vi "PDF Protokoll EPA1065_305 ARN.vi"(8 "error in (no error)":errorcluster caption="Fehler (Eingang, kein Fehler)", 11 "Tabelle":string[][](table)) -> (0 "error out":errorcluster caption="Fehler (Ausgang)")   [LabVIEW 2020, in "EPA 1065.lvlib" / "ARN Test 1065-305.lvlib"]
uses:
  ARN Test 1065-305.lvlib
  T90 1065-308/Ergebnis.ctl
  Seiten/FT-IR/FGV FT-IR Gasliste Aktionen.ctl
  Seiten/FT-IR/FGV FT-IR Aktionen.ctl
  Aktion FGV ARN Daten.ctl
  Aktion FGV Protokoll.ctl
  Seiten/System Einstellungen V2/Aktioen FGV System Konstanten.ctl
  <vilib>/Utility/miscctls.llb/LVPrintingMarginsTypeDef.ctl
  Allgemein/allgemeine Sub-VIs.lvlib
  Seiten/FT-IR/FT-IR.lvlib
  Seiten/System Einstellungen V2/System Einstellungen V2.lvlib
  T90 1065-308/T90 Test 1065-308.lvlib
panel:
  out "Versa Serial number:":string caption="Seriennummer:"
  out "Anlage:":string
  out "Einheit Noise 2":string
  out "Einheit Wiederh. 2":string
  out "Einheit Genauigkeit 2":string
  out "Einheit Noise":string
  out "Einheit Wiederh.":string
  out "Ergebnis 3":T1
  out "Ergebnis 2":T1
  out "Ergebnis 1":T1
  out "Rauschen":string
  out "Rauschen Grenze":string caption="Rauschen:"
  out "Wiederholgenauigkeit":string
  out "Genauigkeit":string
  out "Wiederholgenauigkeit Grenze":string caption="Wiederholgenauigkeit:"
  out "Genauigkeit Grenze":string caption="Genauigkeit:"
  out "Einheit Genauigkeit":string
  out "Tabelle":string[][](table)
  out "Methode (Recipe):":string caption="Methode (Rezept):"
  out "Date & Time:":string caption="Datum & Zeit:"
  out "Accuracy:":string caption="Genauigkeit:"
  out "Gas Bottle Nr.:":string caption="Gasflaschen Nr.:"
  out "T90 Result":waveform(dbl)(graph) caption="T90"
  out "Ergebnis:":string
  out "Konzentration:":string caption="Sollwert:"
  out "Komponente:":string
  out "Bearbeiter:":string
  out "Serial number:":string caption="Seriennummer:"
  out "Messgerät:":string
  # "ANR EPA § 1065.305"
  # "Grenzen"
  # "Ergebnis"
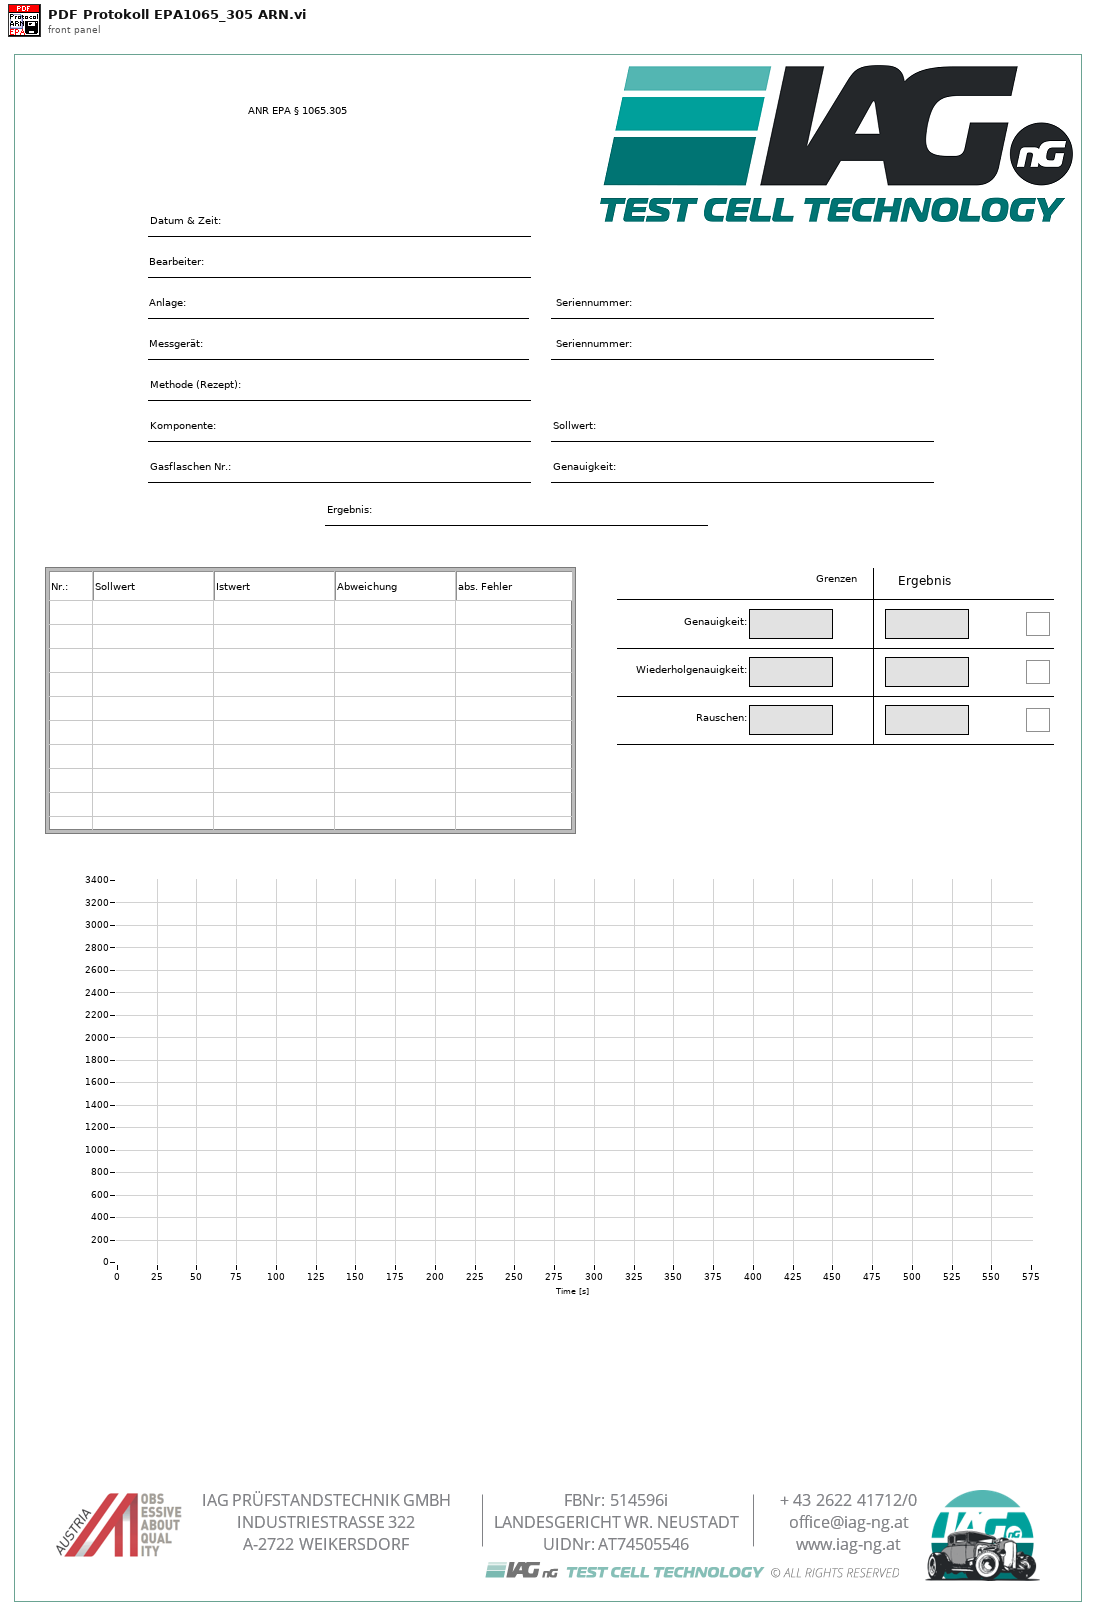
[diagram p1: front panel]
types:
  T1 = typedef "EPA 1065.lvlib/T90 Test 1065-308.lvlib/Ergebnis.ctl" = bool
  T2 = typedef "EPA 1065.lvlib/ARN Test 1065-305.lvlib/Aktion FGV ARN Daten.ctl" = enum16{"Lesen", "laden", "speichern", "ARN Daten", "Rohdaten", "Rohdaten löschen", "Zeitstempel", "SNR Ergebnis"}
  T3 = typedef "FT-IR.lvlib/FGV FT-IR Aktionen.ctl" = enum16{"lesen", "NOG setzen", "NOS setzen", "Initialisieren", "speichern", "ALLES setzen", "FT-IR Spektrum loggen", "Komm Stoppen", "Spektrum LogKonfig"}
  T4 = typedef "FT-IR.lvlib/FGV FT-IR Gasliste Aktionen.ctl" = enum16{"lesen", "Gasliste FT-IR", "Gasliste ausgelesen", "laden", "speichern", "löschen"}
  T5 = typedef "System Einstellungen V2.lvlib/Aktioen FGV System Konstanten.ctl" = enum16{"lesen", "laden", "speichern", "Sprache"}
  T6 = typedef "EPA 1065.lvlib/ARN Test 1065-305.lvlib/Aktion FGV Protokoll.ctl" = enum16{"lesen", "schreiben", "Graph"}
  T7 = enum32{"Portrait", "Landscape", "Rotated Portrait", "Rotated Landscape"}
  T8 = typedef "LVPrintingMarginsTypeDef.ctl" = cluster{"Top":sgl, "Left":sgl, "Bottom":sgl, "Right":sgl, "Measurement System":enum8{"Inches", "cm"}}
  T9 = typedef "EPA 1065.lvlib/ARN Test 1065-305.lvlib/Allgemeine Einstellungen.ctl" = cluster{"Bearbeiter:":string, "Analysator":T10, "Komponente:":u16, "Gasflaschen Nr.:":string, "Accuracy":dbl, "Sollwert":dbl, "Modus":T11, "Pfad:":path, "Textname:":string, "CG Aufschaltzeit:":dbl, "Einheit":string, "N2 Aufschaltzeit:":dbl, "Gasflasche":T12, "Konfig Gasflasche":T13}
  T10 = typedef "System Einstellungen V2.lvlib/Analysatoren.ctl" = string
  T11 = typedef "EPA 1065.lvlib/T90 Test 1065-308.lvlib/Modus.ctl" = u16
  T12 = typedef "System Einstellungen V2.lvlib/Gasflasche Auswahl.ctl" = u16
  T13 = typedef "System Einstellungen V2.lvlib/Konfig Gasflasche.ctl" = bool
  T14 = typedef "String - Ausgabefeld.ctl" = string
  T15 = cluster{"Modell":string, "ProjektNummer":string, "Software Version":string, "Seriennummer":string}
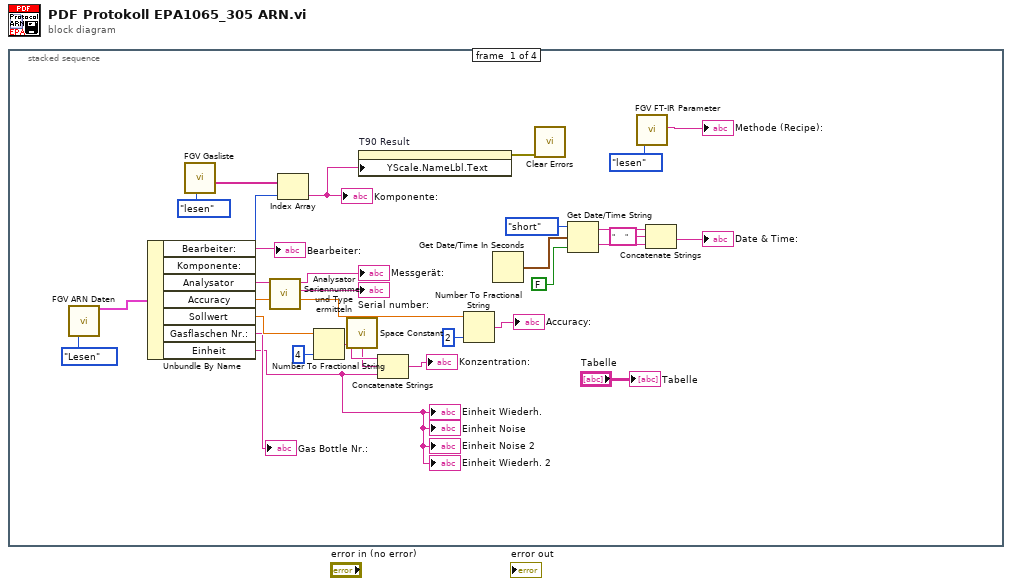
[diagram p0: block diagram]
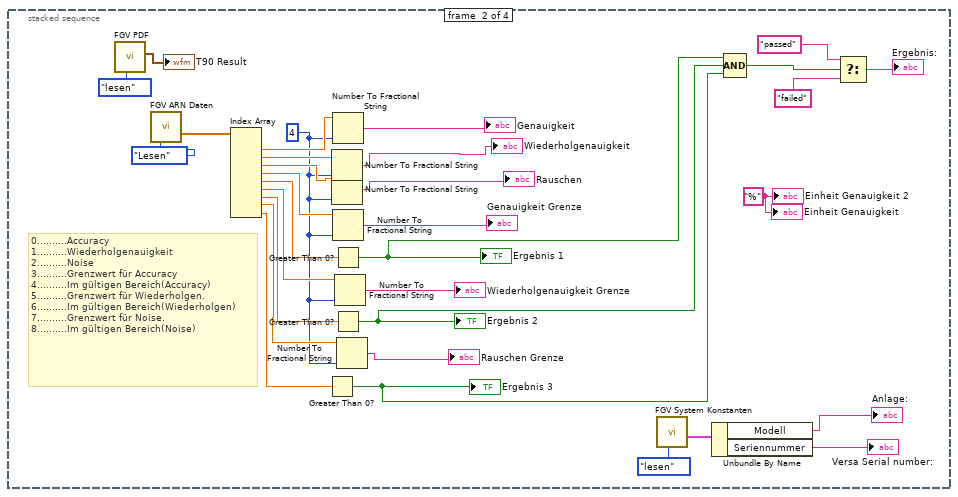
[diagram p2: hidden frame]
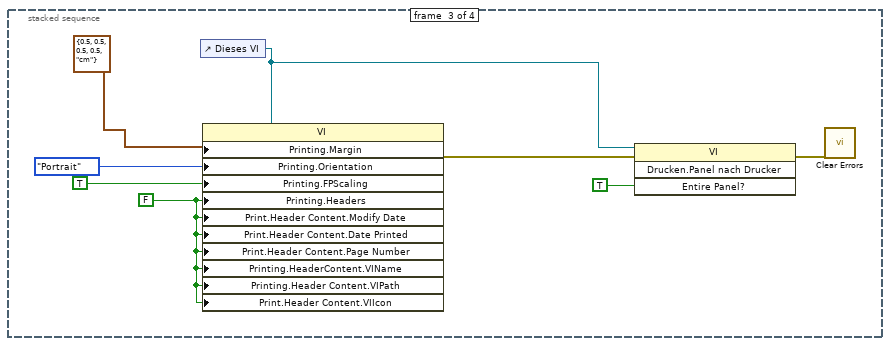
[diagram p3: hidden frame]
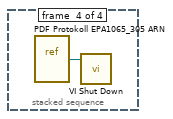
[diagram p4: hidden frame]
diagram:
  n1 = stacked-sequence {
    frame #0 {
      n2 = call "FGV ARN Daten.vi"("Aktion"=Aktion_FGV_ARN_Daten."Lesen") -> ("ARN Konfig Daten"=w6:T9)  [unwired: 9 in, 5 out]
      n3 = Unbundle By Name(w6) -> ("Bearbeiter:"=→"Bearbeiter:":string, "Komponente:"=w21:u16, "Analysator"=w3:T10, "Accuracy"=w18:dbl, "Sollwert"=w14:dbl, "Gasflaschen Nr.:"=→"Gas Bottle Nr.:":string, "Einheit"=w4:string)
      "Einheit Wiederh. 2" <- w4
      "Einheit Noise 2" <- w4
      "Einheit Noise" <- w4
      "Einheit Wiederh." <- w4
      n4 = call "FGV Gasliste.vi"("Aktionen"=FGV_FT-IR_Gasliste_Aktionen."lesen") -> ("Aktuelle Gasliste gesamt"=w22:T14[])  [unwired: 8 in, 2 out]
      n5 = call "Analysator Seriennummer und Type ermitteln.vi"("Analysator"=w3) -> ("Type"=→"Serial number:":string, "Name für Protokoll"=→"Messgerät:":string)  [unwired: 8 in, 1 out]
      n6 = Index Array(array=w22, index=w21) -> (element=w11:T14)
      "Komponente:" <- w11
      n7 = Number To Fractional String(number=w14, precision (6)=i16 4 ("Genauigkeit (6)")) -> (F-format string=w10:string)  [unwired: 2 in]
      n8 = call <vilib>:"Space Constant.vi"() -> ("String"=w8:string)
      n9 = property on="T90 Result" class="SVGraph (strikt)"("YScale.NameLbl.Text"=w11) -> (error out=w12:errorcluster)  [unwired: 2 in, 1 out]
      n10 = Concatenate Strings(w10, w8, w4) -> (→"Konzentration:":string)
      n11 = Number To Fractional String(number=w18, precision (6)=i16 2 ("Genauigkeit (6)")) -> (F-format string=→"Accuracy:":string)  [unwired: 2 in]
      n12 = Get Date/Time In Seconds() -> (seconds since 1Jan1904=w31:timestamp)
      n13 = call <vilib>:"Clear Errors.vi"("error in (no error)"=w12) -> ()  [unwired: 5 in, 2 out]
      n14 = Get Date/Time String(date format (0)=enum16{"short", "long", "abbreviated"}."short" ("Datumsformat (0)"), seconds (now)=w31, want seconds? (F)=FALSE ("Angabe von Sekunden? (F)")) -> (date string=w30:string, time string=w29:string)
      n15 = call "FGV FT-IR Parameter.vi"("Aktion"=FGV_FT-IR_Aktionen."lesen") -> ("Current Recipe"=→"Methode (Recipe):":string)  [unwired: 11 in, 7 out]
      n16 = Concatenate Strings(w30, "     " ("String"), w29) -> (→"Date & Time:":string)
      "Tabelle" <- "Tabelle"
    }
    frame #1 {
      w36 = "%" ("Einheit Genauigkeit 2")
      w47 = i16 4 ("Genauigkeit (6)")
      # "0..........Accuracy\n1..........Wiederholgenauigkeit\n2..........Noise\n3..........Grenzwert für Accuracy\n4..........Im gültigen Bereich(Accuracy)\n5..........Grenzwert für Wiederholgen.\n6..........Im gültigen Bereich(Wiederholgen)\n7..........Grenzwert für Noise.\n8..........Im gültigen Bereich(Noise)"
      n17 = call "FGV PDF.vi"("Aktion"=Aktion_FGV_Protokoll."lesen") -> ("Graph"=→"T90 Result":waveform(dbl))  [unwired: 9 in, 1 out]
      n18 = call "FGV ARN Daten.vi"("Aktion"=Aktion_FGV_ARN_Daten."Lesen") -> ("SNR Ergebnis"=w48:sgl[])  [unwired: 9 in, 5 out]
      n19 = Index Array(array=w48) -> (element #1=w49:sgl, element #2=w50:sgl, element #3=w51:sgl, element #4=w52:sgl, element #5=w53:sgl, element #6=w54:sgl, element #7=w55:sgl, element #8=w56:sgl, element #9=w57:sgl)  [unwired: 9 in]
      n20 = Greater Than 0?(x=w57) -> (x > 0?=w37:bool)
      "Ergebnis 3" <- w37
      n21 = Number To Fractional String(number=w50, precision (6)=w47) -> (F-format string=→"Wiederholgenauigkeit":string)  [unwired: 2 in]
      n22 = Number To Fractional String(number=w51, precision (6)=w47) -> (F-format string=→"Rauschen":string)  [unwired: 2 in]
      n23 = Number To Fractional String(number=w49, precision (6)=w47) -> (F-format string=→"Genauigkeit":string)  [unwired: 2 in]
      n24 = Number To Fractional String(number=w52, precision (6)=w47) -> (F-format string=→"Genauigkeit Grenze":string)  [unwired: 2 in]
      n25 = Greater Than 0?(x=w53) -> (x > 0?=w41:bool)
      "Ergebnis 1" <- w41
      n26 = Greater Than 0?(x=w55) -> (x > 0?=w39:bool)
      "Ergebnis 2" <- w39
      n27 = Number To Fractional String(number=w54, precision (6)=w47) -> (F-format string=→"Wiederholgenauigkeit Grenze":string)  [unwired: 2 in]
      n28 = Number To Fractional String(number=w56, precision (6)=w47) -> (F-format string=→"Rauschen Grenze":string)  [unwired: 2 in]
      n29 = call "FGV System Konstanten.vi"("Aktionen"=Aktioen_FGV_System_Konstanten."lesen") -> ("Cluster out"=w34:T15)  [unwired: 6 in, 4 out]
      n30 = Unbundle By Name(w34) -> ("Modell"=→"Anlage:":string, "Seriennummer"=→"Versa Serial number:":string)
      n31 = Compound Arithmetic op=AND ("Mehrfacharithmetik")(w41, w39, w37) -> (w60:bool)
      n32 = Select(t="passed", s=w60, f="failed") -> (s? t:f=→"Ergebnis:":string)
      "Einheit Genauigkeit 2" <- w36
      "Einheit Genauigkeit" <- w36
    }
    frame #2 {
      w67 = FALSE ("Drucken:Kopfzeilen?")
      n33 = control-ref of="Dieses VI"() -> (w64:refnum<vi>)
      n34 = property class="VI"(reference=w64, "Printing.Margin"=T8 {"Top"=0.5, "Left"=0.5, "Bottom"=0.5, "Right"=0.5, "Measurement System"=enum."cm"} ("Drucken:Ränder"), "Printing.Orientation"=T7."Portrait" ("Drucken:Seitenausrichtung"), "Printing.FPScaling"=TRUE ("Drucken:Frontpanel-Skalierung?"), "Printing.Headers"=w67, "Print.Header Content.Modify Date"=w67, "Print.Header Content.Date Printed"=w67, "Print.Header Content.Page Number"=w67, "Printing.HeaderContent.VIName"=w67, "Printing.Header Content.VIPath"=w67, "Print.Header Content.VIIcon"=w67) -> (error out=w71:errorcluster)  [unwired: 1 in, 1 out]
      n35 = invoke class="VI" method="Drucken.Panel nach Drucker"(reference=w64, error in=w71, "Entire Panel?"=TRUE ("Abschnittskopfzeilen?")) -> (error out=w65:errorcluster)  [unwired: 1 in, 3 out]
      n36 = call <vilib>:"Clear Errors.vi"("error in (no error)"=w65) -> ()  [unwired: 5 in, 2 out]
    }
    frame #3 {
      n37 = vi-ref "PDF Protokoll EPA1065_305 ARN.vi"() -> (w72:refnum<vi>)
      n38 = call "VI Shut Down.vi"("VI Referenz"=w72) -> ()  [unwired: 11 in]
    }
  }
